vi "ServoTime.vi"() -> ()   [LabVIEW 2026]
panel:
  out "Meter":dbl(knob) scale=0.0..10.0
  out "?":string
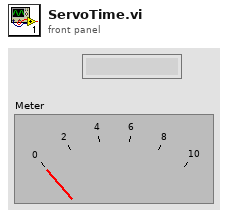
[diagram p1: front panel]
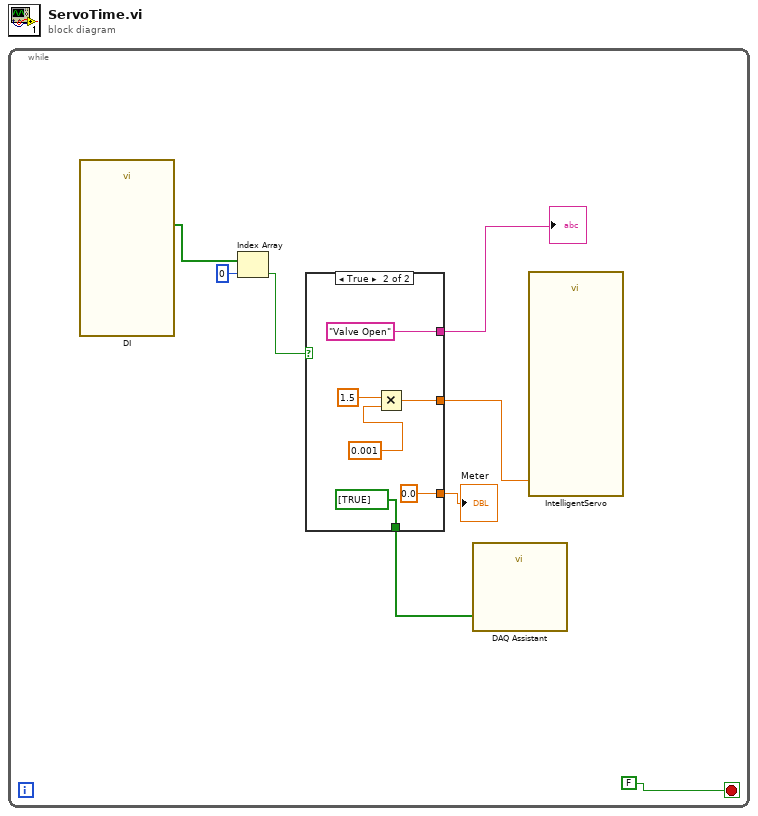
[diagram p0: block diagram]
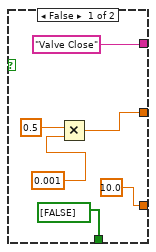
[diagram p2: hidden frame]
diagram:
  n1 = while {
    stop <- FALSE stop-if-true
    n2 = call "DI.vi"() -> ("data"=w8:bool[])  [unwired: 17 in, 2 out]
    n3 = Index Array(array=w8, index=0) -> (element=w7:bool)
    n4 = case shown="True" w7 {
      tunnel: [w12 w18] -> w5
      tunnel: [bool[] [FALSE] ("data") bool[] [TRUE] ("data")] -> w3
      tunnel: ["Valve Close" "Valve Open"] -> w2
      tunnel: [10.0 0.0] -> w1
      frame False {
        n5 = Multiply(x=0.5, y=0.001) -> (x*y=w12:dbl)
      }
      frame True {
        n6 = Multiply(x=1.5, y=0.001) -> (x*y=w18:dbl)
      }
    }
    "?" <- w2
    "Meter" <- w1
    n7 = call "DAQ Assistant"("data"=w3) -> ()  [unwired: 17 in, 2 out]
    n8 = call "IntelligentServo.vi"("timeout (s) 2"=w5) -> ()  [unwired: 17 in, 2 out]
  }
